vi "Wait Timer.vi"(3 "Boolean In":bool, 4 "Timer":u32) -> (5 "Boolean Out":bool)   [LabVIEW 2014]
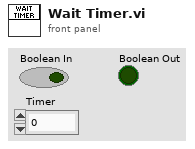
[diagram p1: front panel]
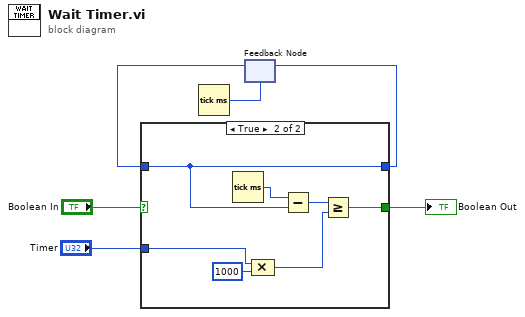
[diagram p0: block diagram]
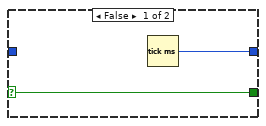
[diagram p2: hidden frame]
diagram:
  n1 = Tick Count (ms)() -> (millisecond timer value=w1:u32)
  n2 = feedback #1(w1) -> (w3:u32)
  n3 = case shown="True" "Boolean In" {
    selector: "Boolean In" -> [w8 _]
    tunnel: "Timer" -> [_ w13]
    tunnel: [w7 w9] -> w4
    tunnel: w3 -> [_ w9]
    tunnel: [w8 w10] -> w2
    frame False {
      n4 = Tick Count (ms)() -> (millisecond timer value=w7:u32)
    }
    frame True {
      n5 = Tick Count (ms)() -> (millisecond timer value=w15:u32)
      n6 = Compound Arithmetic op=MULTIPLY(w13, u32 1000 ("value")) -> (w11:u32)
      n7 = Subtract(x=w15, y=w9) -> (x-y=w14:u32)
      n8 = Greater Or Equal?(x=w14, y=w11) -> (x >= y?=w10:bool)
    }
  }
  "Boolean Out" <- w2
  n9 = feedback-in #1(w4) -> ()
